vi "外观 1.vi"(0 "Data In":T4 caption="数据输入", 2 "Display State In":T2 caption="显示状态输入", 3 "Container State":T3 caption="容器状态") -> (6 "Data Out":T4 caption="数据输出", 7 "Display State Out":T2 caption="显示状态输出", 8 "Action":T1 caption="动作")   [LabVIEW 2016, in "主画面菜单.xctl"]
uses:
  <vilib>/_xctls/Container State.ctl
  <vilib>/_xctls/Action.ctl
  <vilib>/_xctls/XControlSupport.lvlib
panel:
  in  "单选按钮":enum32{"首页", "数据查询", "运维调试", "系统设置"}(radio)
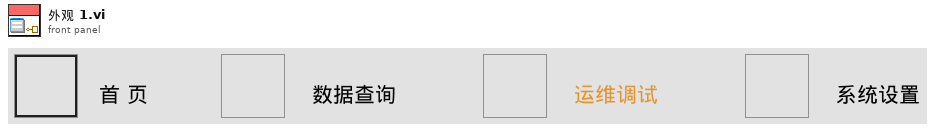
[diagram p1: front panel]
types:
  T1 = typedef "XControlSupport.lvlib/Action.ctl" = cluster{"Data Changed?":bool, "State Changed?":bool, "Action Name":string}
  T2 = typedef "主画面菜单.xctl/状态 1.ctl" = cluster{"Numeric":dbl}
  T3 = typedef "XControlSupport.lvlib/Container State.ctl" = cluster{"Indicator?":bool, "Run Mode?":bool, " Refnum":refnum<vi>}
  T4 = typedef "主画面菜单.xctl/数据 1.ctl" = enum32{"首页", "数据查询", "运维调试", "系统设置"}
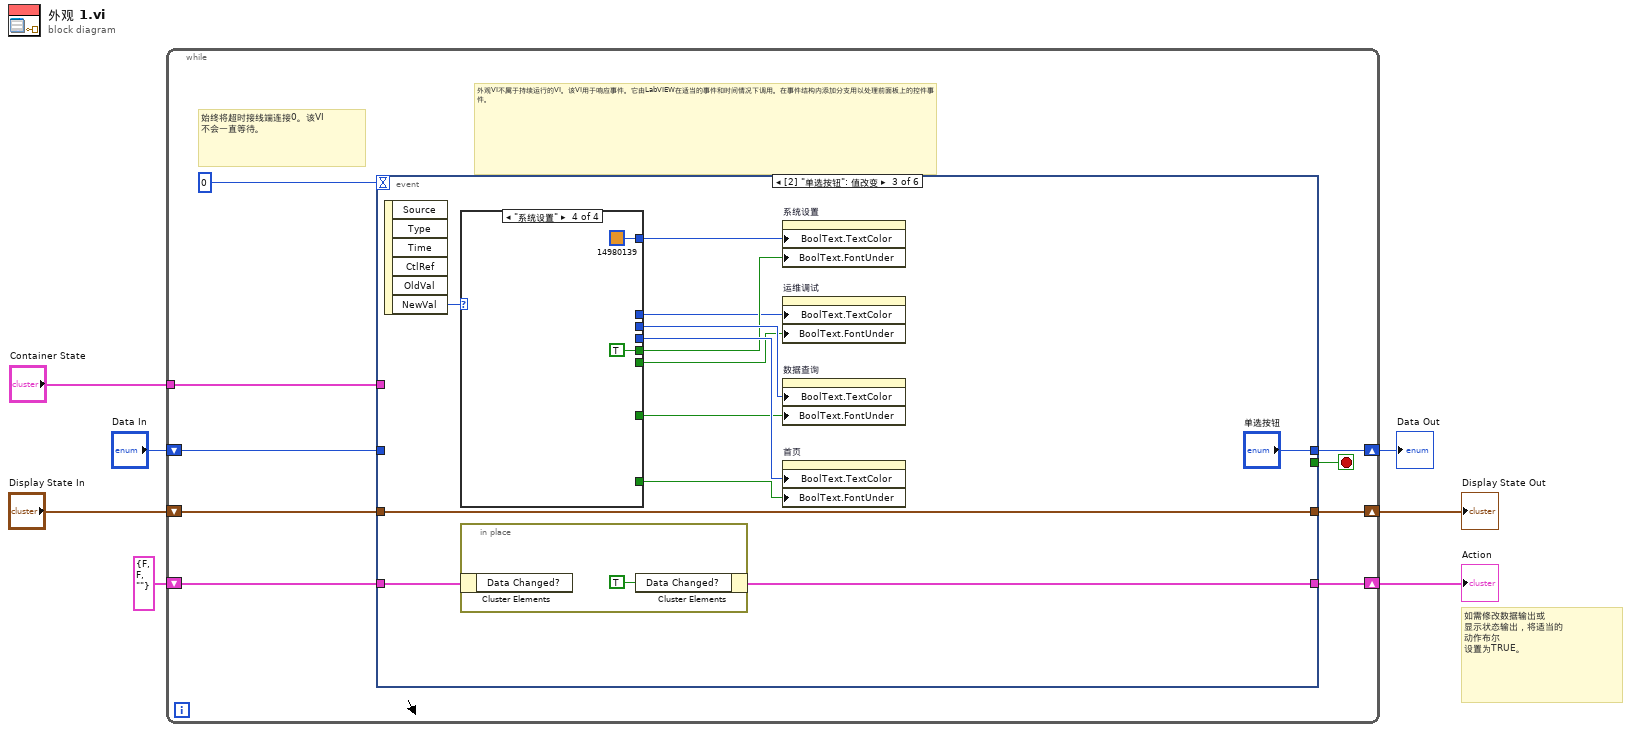
[diagram p0: block diagram]
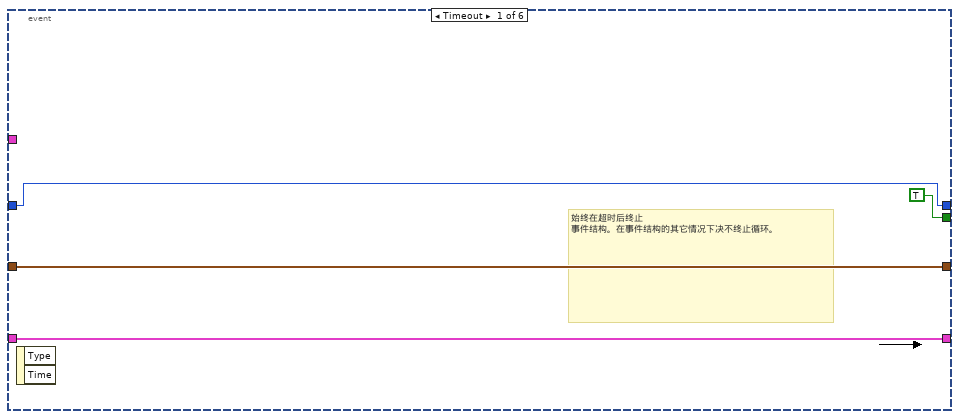
[diagram p2: hidden frame]
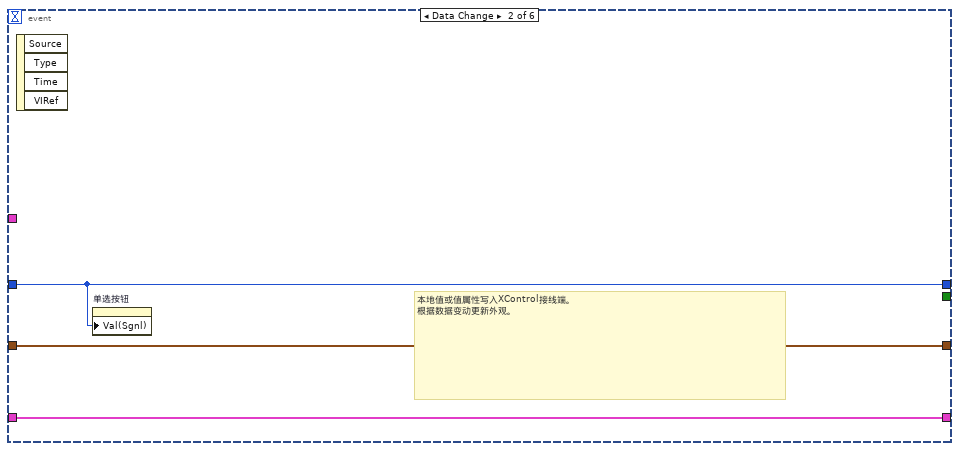
[diagram p3: hidden frame]
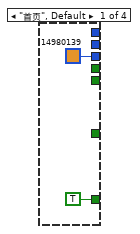
[diagram p4: hidden frame]
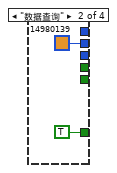
[diagram p5: hidden frame]
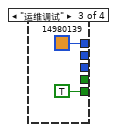
[diagram p6: hidden frame]
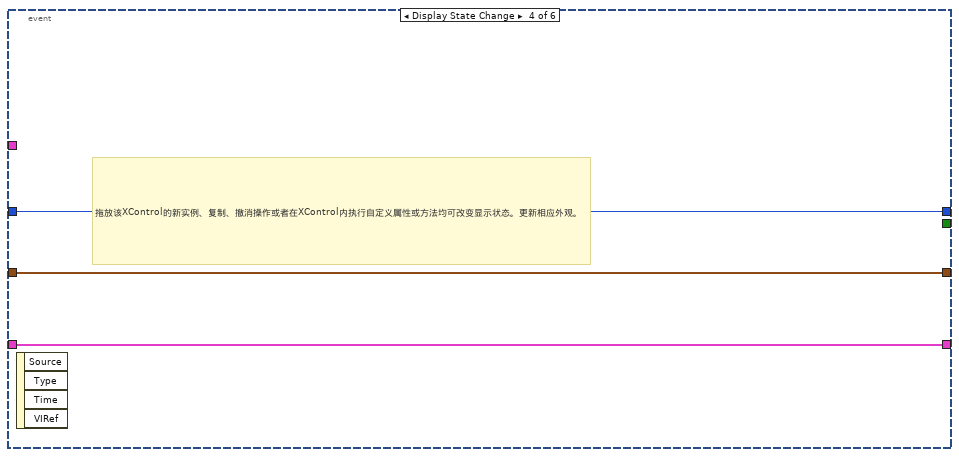
[diagram p7: hidden frame]
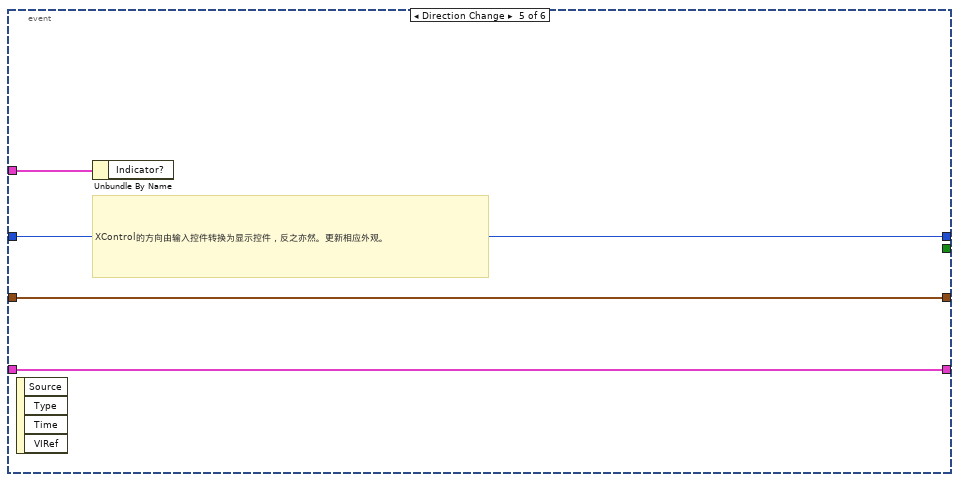
[diagram p8: hidden frame]
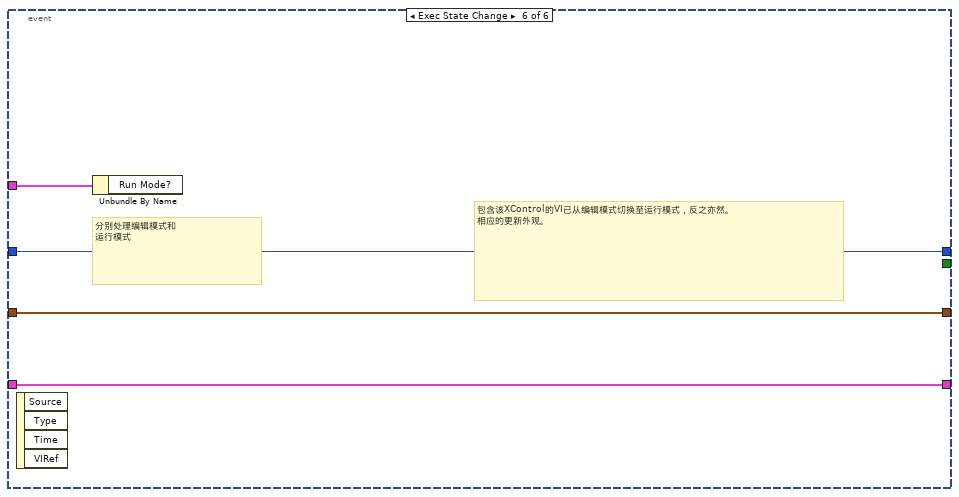
[diagram p9: hidden frame]
diagram:
  # "如需修改数据输出或\n显示状态输出，将适当的\n动作布尔\n设置为TRUE。"
  n1 = while {
    shift-right: [w15] -> w4
    shift-left: "Display State In" -> [w16]
    tunnel: "Container State" -> [w12]
    shift-right: [w10] -> w7
    shift-left: "Data In" -> [w11]
    shift-right: [w8] -> w2
    shift-left: T1 {"Data Changed?"=FALSE, "State Changed?"=FALSE, "Action Name"=""} ("Action") -> [w9]
    stop <- w14 stop-if-true
    # "外观VI不属于持续运行的VI。该VI用于响应事件。它由LabVIEW在适当的事件和时间情况下调用。在事件结构内添加分支用以处理前面板上的控件事件。"
    # "始终将超时接线端连接0。该VI\n不会一直等待。"
    n2 = event shown="[2] \"单选按钮\": 值改变" {
      selector: _ -> [_ _ _ _ _ _]
      dyn-events: _ -> [_ _ _ _ _ _]
      timeout: 0 -> [_ _ _ _ _ _]
      tunnel: w16 -> [w18 w23 w36 w48 w51 w55]
      tunnel: [w18 w23 w36 w48 w51 w55] -> w15
      tunnel: [TRUE _ _ _ _ _] -> w14
      tunnel: w12 -> [_ _ _ _ w52 w56]
      tunnel: w11 -> [w17 w21 _ w47 w50 w54]
      tunnel: [w17 w21 "单选按钮" w47 w50 w54] -> w10
      tunnel: [w19 w22 w34 w46 w49 w53] -> w8
      tunnel: w9 -> [w19 w22 w35 w46 w49 w53]
      event Timeout {
        # "始终在超时后终止\n事件结构。在事件结构的其它情况下决不终止循环。"
        n3 = event-data() -> ()  [unwired: 1 in, 2 out]
      }
      event Data Change {
        # "本地值或值属性写入XControl接线端。\n根据数据变动更新外观。"
        n4 = event-data() -> ()  [unwired: 1 in, 4 out]
        n5 = property on="单选按钮" class="RadioBtnsControl (严格)"("Val(Sgnl)"=w21) -> ()  [unwired: 2 in, 2 out]
      }
      event "单选按钮": Value Change {
        n6 = event-data() -> ("NewVal"=w24:enum32{"首页", "数据查询", "运维调试", "系统设置"})  [unwired: 1 in, 5 out]
        n7 = case shown="\"系统设置\"" w24 {
          tunnel: [TRUE ("布尔文本.字体:下划线") _ _ _] -> w32
          tunnel: [u32 14980139 _ _ _] -> w31
          tunnel: [_ TRUE ("布尔文本.字体:下划线") _ _] -> w30
          tunnel: [_ u32 14980139 _ _] -> w29
          tunnel: [_ _ u32 14980139 _] -> w25
          tunnel: [_ _ TRUE ("布尔文本.字体:下划线") _] -> w28
          tunnel: [_ _ _ u32 14980139] -> w27
          tunnel: [_ _ _ TRUE ("布尔文本.字体:下划线")] -> w26
          frame "首页", Default {
          }
          frame "数据查询" {
          }
          frame "运维调试" {
          }
          frame "系统设置" {
          }
        }
        n8 = in-place {
          n9 = in-place-cluster #1(w35) -> ()  [unwired: 1 out]
          n10 = in-place-cluster #1("Data Changed?"=TRUE) -> (w34:T1)
        }
        n11 = property on="系统设置" class="Bool (严格)"("BoolText.TextColor"=w27, "BoolText.FontUnder"=w26) -> ()  [unwired: 2 in, 2 out]
        n12 = property on="运维调试" class="Bool (严格)"("BoolText.TextColor"=w25, "BoolText.FontUnder"=w28) -> ()  [unwired: 2 in, 2 out]
        n13 = property on="数据查询" class="Bool (严格)"("BoolText.TextColor"=w29, "BoolText.FontUnder"=w30) -> ()  [unwired: 2 in, 2 out]
        n14 = property on="首页" class="Bool (严格)"("BoolText.TextColor"=w31, "BoolText.FontUnder"=w32) -> ()  [unwired: 2 in, 2 out]
      }
      event Display State Change {
        # "拖放该XControl的新实例、复制、撤消操作或者在XControl内执行自定义属性或方法均可改变显示状态。更新相应外观。"
        n15 = event-data() -> ()  [unwired: 1 in, 4 out]
      }
      event Direction Change {
        # "XControl的方向由输入控件转换为显示控件，反之亦然。更新相应外观。"
        n16 = event-data() -> ()  [unwired: 1 in, 4 out]
        n17 = Unbundle By Name(w52) -> ()  [unwired: 1 out]
      }
      event Exec State Change {
        # "包含该XControl的VI已从编辑模式切换至运行模式，反之亦然。\n相应的更新外观。"
        # "分别处理编辑模式和\n运行模式"
        n18 = event-data() -> ()  [unwired: 1 in, 4 out]
        n19 = Unbundle By Name(w56) -> ()  [unwired: 1 out]
      }
    }
  }
  "Display State Out" <- w4
  "Data Out" <- w7
  "Action" <- w2
